vi "EllipRegionConstraint_IsPoseInRegion.vi"(10 "statePose":T4={"TRANSLATION"={"X"=0.0, "Y"=0.0}, "ROTATION"={"VALUE"=0.0, "COS"=1.0, "SIN"=0.0}} {"ROTATION"."SIN" format="%13.4f"; "ROTATION"."COS" format="%13.4f"; "ROTATION"."VALUE" format="%13.4f"; "TRANSLATION"."Y" format="%14.3f"; "TRANSLATION"."X" format="%14.3f"}, 11 "ELLIP_REGION_CONSTRAINT":T1={"Center"={"X"=0.0, "Y"=0.0}, "Radii"={"X"=0.0, "Y"=0.0}, "Constraint"=variant, "Constraint Type"=enum."DIFF DRIVE KINEMATICS", "IM UNIQUE"=FALSE} {"Radii"."Y" format="%14.3f"; "Radii"."X" format="%14.3f"; "Center"."Y" format="%14.3f"; "Center"."X" format="%14.3f"}) -> (3 "PoseInRegion":bool)   [LabVIEW 2019, in "Trajectory_Library.lvlib"]
doc: "Determines if the robot pose is within the defined region.\n\nParameters:\n - Elliptical Region Constraint -- Constraint data cluster.\n - statePose - current traj state Pose\n\nReturns\n - PoseInRegion -- TRUE if pose is within the region."
uses:
  Trajectory_Library.lvlib
  TypeDef/TRANSLATION2D.ctl
  TypeDef/ROTATION2D.ctl
  TypeDef/POSE2D.ctl
  Enum/TRAJ_CONSTRAINT_TYPES_ENUM.ctl
  TypeDef/TRAJ_CONSTRAINT_ELLIP_REGION.ctl
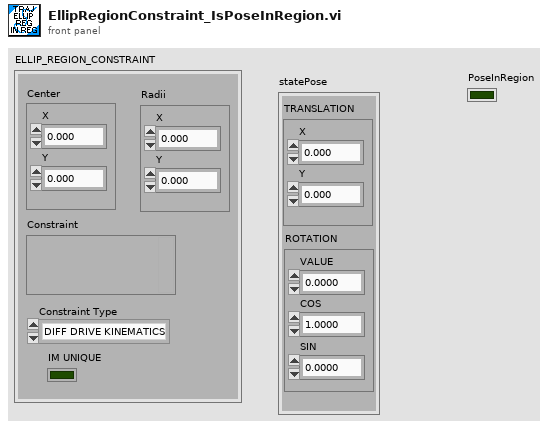
[diagram p1: front panel]
types:
  T1 = typedef "Trajectory_Library.lvlib/TRAJ_CONSTRAINT_ELLIP_REGION.ctl" = cluster{"Center":T2, "Radii":T2, "Constraint":variant, "Constraint Type":T3, "IM UNIQUE":bool}
  T2 = typedef "Trajectory_Library.lvlib/TRANSLATION2D.ctl" = cluster{"X":dbl, "Y":dbl}
  T3 = typedef "Trajectory_Library.lvlib/TRAJ_CONSTRAINT_TYPES_ENUM.ctl" = enum16{"UNDEFINED", "DIFF DRIVE KINEMATICS", "DIFF DRIVE VOLTAGE", "CENTRIPITAL ACCEL", "MECA DRIVE KINEMATICS", "SWERVE DRIVE KINEMATICS", "MAXIMUM VELOCITY", "ELLIPTICAL REGION", "RECTANGULAR REGION"}
  T4 = typedef "Trajectory_Library.lvlib/POSE2D.ctl" = cluster{"TRANSLATION":T2, "ROTATION":T5}
  T5 = typedef "Trajectory_Library.lvlib/ROTATION2D.ctl" = cluster{"VALUE":dbl, "COS":dbl, "SIN":dbl}
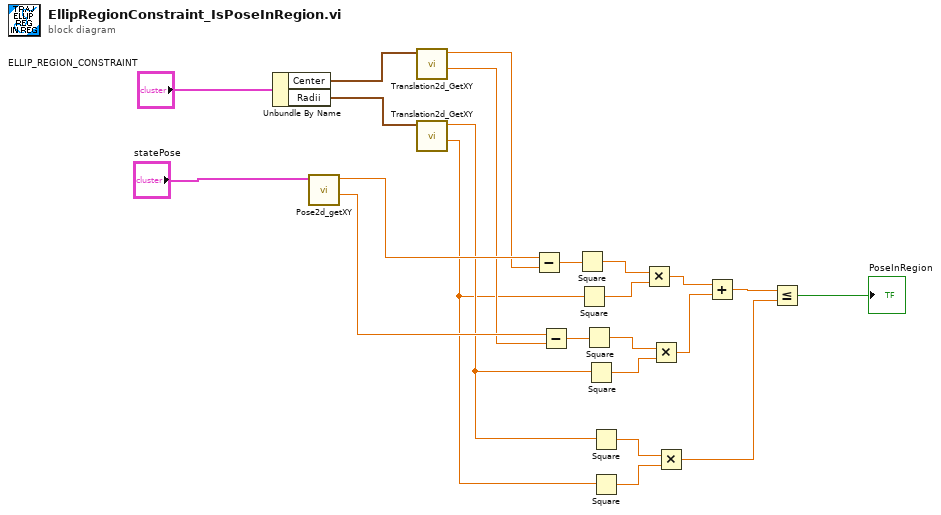
[diagram p0: block diagram]
diagram:
  n1 = Unbundle By Name("ELLIP_REGION_CONSTRAINT") -> ("Center"=w22:T2, "Radii"=w21:T2)
  n2 = call "Pose2d_getXY.vi"("in POSE"="statePose") -> ("Y"=w11:dbl, "X"=w19:dbl)  [unwired: 9 in]
  n3 = call "Translation2d_GetXY.vi"("In Translation"=w22) -> ("Y"=w10:dbl, "X"=w18:dbl)  [unwired: 9 in]
  n4 = call "Translation2d_GetXY.vi"("In Translation"=w21) -> ("Y"=w5:dbl, "X"=w6:dbl)  [unwired: 9 in]
  n5 = Subtract(x=w19, y=w18) -> (x-y=w17:dbl)
  n6 = Subtract(x=w11, y=w10) -> (x-y=w14:dbl)
  n7 = Square(x=w17) -> (x^2=w16:dbl)
  n8 = Square(x=w5) -> (x^2=w15:dbl)
  n9 = Square(x=w14) -> (x^2=w13:dbl)
  n10 = Square(x=w6) -> (x^2=w12:dbl)
  n11 = Square(x=w6) -> (x^2=w4:dbl)
  n12 = Square(x=w5) -> (x^2=w3:dbl)
  n13 = Multiply(x=w16, y=w15) -> (x*y=w9:dbl)
  n14 = Multiply(x=w13, y=w12) -> (x*y=w8:dbl)
  n15 = Multiply(x=w4, y=w3) -> (x*y=w2:dbl)
  n16 = Add(x=w9, y=w8) -> (x+y=w7:dbl)
  n17 = Less Or Equal?(x=w7, y=w2) -> (x <= y?=→"PoseInRegion":bool)
